vi "Timed Test.vi"() -> ()   [LabVIEW 2017]
uses:
  122af3c8-ed90-4da6-ba5e-d7198250e946.vi
  String Subset.vi
  Parsing/Parse Full Path or Item Name.vi
  Offset/Find Item Locations by Path.vi
  JSON text to Variant.vi
  JSONtext.lvlib
panel:
  out "time":dbl format="%#_3p"
  out "value":string
  out "Offsets":i32[](array[numeric])
  out "<JSON>":string[](array[string]) caption="<JSON>Items"
  out "Waveform Chart":dbl(graph)
  out "time/char":dbl format="%#_3p"
  out "Offset past Value":i32
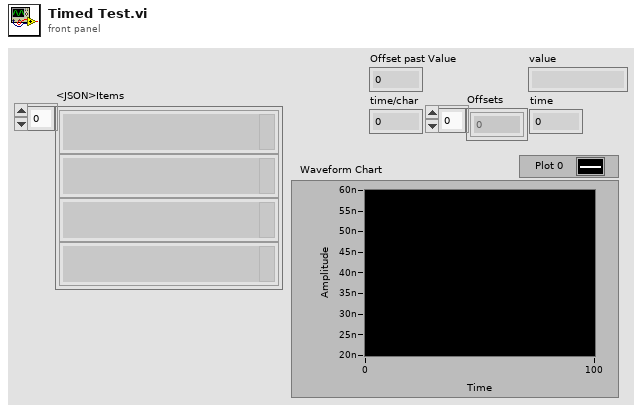
[diagram p1: front panel]
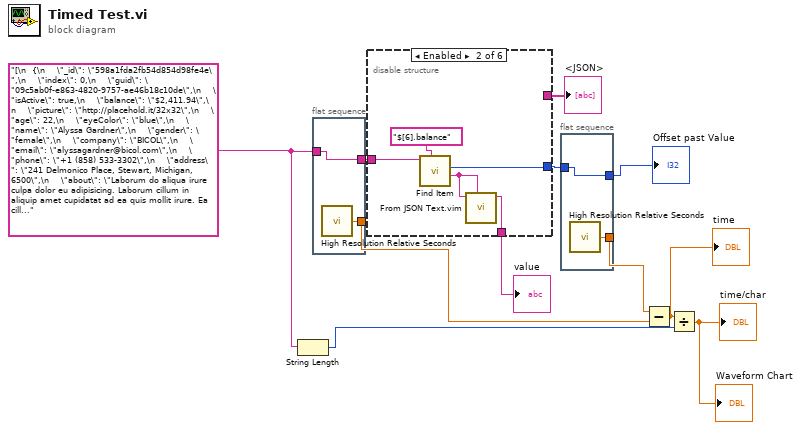
[diagram p0: block diagram]
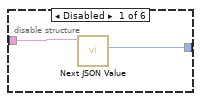
[diagram p2: hidden frame]
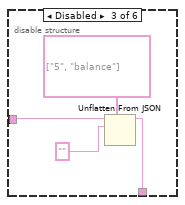
[diagram p3: hidden frame]
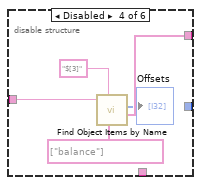
[diagram p4: hidden frame]
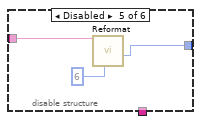
[diagram p5: hidden frame]
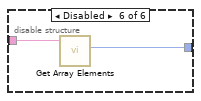
[diagram p6: hidden frame]
diagram:
  w6 = "[\n  {\n    \"_id\": \"598a1fda2fb54d854d98fe4e\",\n    \"index\": 0,\n    \"guid\": \"09c5ab0f-e863-4820-9757-ae46b18c10de\",\n    \"isActive\": true,\n    \"balance\": \"$2,411.94\",\n    \"picture\": \"http://placehold.it/32x32\",\n    \"age\": 22,\n    \"eyeColor\": \"blue\",\n    \"name\": \"Alyssa Gardner\",\n    \"gender\": \"female\",\n    \"company\": \"BICOL\",\n    \"email\": \"alyssagardner@bicol.com\",\n    \"phone\": \"+1 (858) 533-3302\",\n    \"address\": \"241 Delmonico Place, Stewart, Michigan, 6500\",\n    \"about\": \"Laborum do aliqua irure culpa dolor eu adipisicing. Laborum cillum in aliquip amet cupidatat ad ea quis mollit irure. Ea cillum exercitation nulla Lorem exercitation velit ad reprehenderit sint sint cupidatat elit reprehenderit. Incididunt aute tempor culpa ea sunt do sunt est deserunt deserunt eiusmod irure amet. Pariatur voluptate ea quis cupidatat non sit.\\r\\n\",\n    \"registered\": \"2016-12-13T10:56:52 -00:00\",\n    \"latitude\": -9.98155,\n    \"longitude\": -80.627111,\n    \"tags\": [\n      \"ad\",\n      \"cillum\",\n      \"est\",\n      \"et\",\n      \"deserunt\",\n      \"aliquip\",\n      \"cillum\"\n    ],\n    \"friends\": [\n      {\n        \"id\": 0,\n        \"name\": \"Karyn Weber\"\n      },\n      {\n        \"id\": 1,\n        \"name\": \"King Acevedo\"\n      },\n      {\n        \"id\": 2,\n        \"name\": \"Tanisha Rodgers\"\n      }\n    ],\n    \"greeting\": \"Hello, Alyssa Gardner! You have 6 unread messages.\",\n    \"favoriteFruit\": \"strawberry\"\n  },\n  {\n    \"_id\": \"598a1fda30b27ecb1964e718\",\n    \"index\": 1,\n    \"guid\": \"b7cddb7f-e542-4f41-b26c-7ddbecc986b3\",\n    \"isActive\": false,\n    \"balance\": \"$1,317.36\",\n    \"picture\": \"http://placehold.it/32x32\",\n    \"age\": 25,\n    \"eyeColor\": \"blue\",\n    \"name\": \"Skinner Andrews\",\n    \"gender\": \"male\",\n    \"company\": \"REMOLD\",\n    \"email\": \"skinnerandrews@remold.com\",\n    \"phone\": \"+1 (953) 523-2141\",\n    \"address\": \"515 Balfour Place, Gratton, Tennessee, 1793\",\n    \"about\": \"Nisi deserunt consectetur dolore reprehenderit ipsum dolore voluptate tempor nostrud est labore. Laborum ullamco do irure duis sunt sit quis consectetur dolore quis. Et veniam eu ad dolor. Anim incididunt tempor adipisicing elit veniam. Laboris esse amet pariatur pariatur aliqua ea dolore sunt dolor anim aliqua elit. Velit ipsum commodo deserunt esse aliquip sit.\\r\\n\",\n    \"registered\": \"2016-12-25T06:53:25 -00:00\",\n    \"latitude\": 72.774284,\n    \"longitude\": -22.688458,\n    \"tags\": [\n      \"dolore\",\n      \"nulla\",\n      \"deserunt\",\n      \"laboris\",\n      \"excepteur\",\n      \"eiusmod\",\n      \"ad\"\n    ],\n    \"friends\": [\n      {\n        \"id\": 0,\n        \"name\": \"Barron Rios\"\n      },\n      {\n        \"id\": 1,\n        \"name\": \"Roy Roy\"\n      },\n      {\n        \"id\": 2,\n        \"name\": \"Tonia Gates\"\n      }\n    ],\n    \"greeting\": \"Hello, Skinner Andrews! You have 5 unread messages.\",\n    \"favoriteFruit\": \"strawberry\"\n  },\n  {\n    \"_id\": \"598a1fdafd338fee73c75cc9\",\n    \"index\": 2,\n    \"guid\": \"e12f53e7-ffe2-40da-87a4-988a62c535d3\",\n    \"isActive\": true,\n    \"balance\": \"$3,792.67\",\n    \"picture\": \"http://placehold.it/32x32\",\n    \"age\": 21,\n    \"eyeColor\": \"green\",\n    \"name\": \"Lillie Spears\",\n    \"gender\": \"female\",\n    \"company\": \"KNEEDLES\",\n    \"email\": \"lilliespears@kneedles.com\",\n    \"phone\": \"+1 (946) 421-3701\",\n    \"address\": \"744 Dearborn Court, Brandywine, Massachusetts, 8302\",\n    \"about\": \"Dolor ad est cupidatat velit excepteur sunt. Id amet laborum nulla id magna deserunt nostrud et Lorem. Laboris amet tempor est cupidatat ullamco. Dolore Lorem aute duis quis sint in. Proident sunt laboris consectetur quis.\\r\\n\",\n    \"registered\": \"2016-01-29T12:32:53 -00:00\",\n    \"latitude\": -72.39395,\n    \"longitude\": -125.497614,\n    \"tags\": [\n      \"voluptate\",\n      \"sunt\",\n      \"et\",\n      \"amet\",\n      \"ea\",\n      \"anim\",\n      \"nisi\"\n    ],\n    \"friends\": [\n      {\n        \"id\": 0,\n        \"name\": \"Guzman Mcmahon\"\n      },\n      {\n        \"id\": 1,\n        \"name\": \"Craig Sampson\"\n      },\n      {\n        \"id\": 2,\n        \"name\": \"Gilliam Joseph\"\n      }\n    ],\n    \"greeting\": \"Hello, Lillie Spears! You have 5 unread messages.\",\n    \"favoriteFruit\": \"strawberry\"\n  },\n  {\n    \"_id\": \"598a1fdaae68ee444817bd5d\",\n    \"index\": 3,\n    \"guid\": \"896b1e41-bfd2-4e40-ac6f-ac9896540f87\",\n    \"isActive\": false,\n    \"balance\": \"$2,127.27\",\n    \"picture\": \"http://placehold.it/32x32\",\n    \"age\": 31,\n    \"eyeColor\": \"brown\",\n    \"name\": \"Massey Lopez\",\n    \"gender\": \"male\",\n    \"company\": \"BOLAX\",\n    \"email\": \"masseylopez@bolax.com\",\n    \"phone\": \"+1 (890) 530-3697\",\n    \"address\": \"130 National Drive, Eagleville, Oregon, 7451\",\n    \"about\": \"Excepteur elit consectetur Lorem occaecat culpa eu consequat reprehenderit dolore irure ullamco eiusmod mollit. Ut in aliquip dolor occaecat laborum officia veniam cillum. Consequat enim minim tempor culpa adipisicing et adipisicing aliqua esse minim fugiat. Magna in aute sint officia pariatur culpa. Labore exercitation quis laborum ipsum cillum incididunt dolor nostrud deserunt pariatur do sunt. Officia tempor consectetur sunt aliquip cillum nostrud do Lorem in. Sunt commodo minim officia nulla fugiat qui anim.\\r\\n\",\n    \"registered\": \"2016-06-20T11:25:17 -01:00\",\n    \"latitude\": -25.916761,\n    \"longitude\": -176.019318,\n    \"tags\": [\n      \"nisi\",\n      \"nisi\",\n      \"aliqua\",\n      \"nostrud\",\n      \"aliquip\",\n      \"mollit\",\n      \"cillum\"\n    ],\n    \"friends\": [\n      {\n        \"id\": 0,\n        \"name\": \"Florine Hubbard\"\n      },\n      {\n        \"id\": 1,\n        \"name\": \"Harper Peterson\"\n      },\n      {\n        \"id\": 2,\n        \"name\": \"Hayes Kaufman\"\n      }\n    ],\n    \"greeting\": \"Hello, Massey Lopez! You have 8 unread messages.\",\n    \"favoriteFruit\": \"banana\"\n  },\n  {\n    \"_id\": \"598a1fda5ee0d6fed3630e62\",\n    \"index\": 4,\n    \"guid\": \"8e1a25a0-83eb-45b2-9e18-c4b03a903295\",\n    \"isActive\": true,\n    \"balance\": \"$1,882.49\",\n    \"picture\": \"http://placehold.it/32x32\",\n    \"age\": 26,\n    \"eyeColor\": \"brown\",\n    \"name\": \"Ginger Black\",\n    \"gender\": \"female\",\n    \"company\": \"KROG\",\n    \"email\": \"gingerblack@krog.com\",\n    \"phone\": \"+1 (924) 450-3688\",\n    \"address\": \"843 Jackson Place, Greenwich, Puerto Rico, 8966\",\n    \"about\": \"Nostrud tempor quis elit nulla consectetur. Reprehenderit voluptate enim ea aliquip minim commodo proident ipsum commodo ex. Commodo nisi nulla magna amet. Officia minim cillum minim nostrud eiusmod tempor ut cillum cillum culpa. Non do reprehenderit esse consectetur aliquip. Ipsum excepteur esse veniam id nulla sunt enim nulla reprehenderit elit non reprehenderit fugiat dolore.\\r\\n\",\n    \"registered\": \"2016-03-21T08:14:28 -00:00\",\n    \"latitude\": 16.438889,\n    \"longitude\": -11.148876,\n    \"tags\": [\n      \"commodo\",\n      \"ipsum\",\n      \"exercitation\",\n      \"est\",\n      \"culpa\",\n      \"do\",\n      \"anim\"\n    ],\n    \"friends\": [\n      {\n        \"id\": 0,\n        \"name\": \"Taylor Ball\"\n      },\n      {\n        \"id\": 1,\n        \"name\": \"Irma Guerrero\"\n      },\n      {\n        \"id\": 2,\n        \"name\": \"Allison Fitzpatrick\"\n      }\n    ],\n    \"greeting\": \"Hello, Ginger Black! You have 6 unread messages.\",\n    \"favoriteFruit\": \"strawberry\"\n  },\n  {\n    \"_id\": \"598a1fdab7c3311e6bd5eb22\",\n    \"index\": 5,\n    \"guid\": \"81b72db8-8d6a-4430-a934-c8454fbade9b\",\n    \"isActive\": true,\n    \"balance\": \"$2,347.48\",\n    \"picture\": \"http://placehold.it/32x32\",\n    \"age\": 23,\n    \"eyeColor\": \"blue\",\n    \"name\": \"Hobbs Rocha\",\n    \"gender\": \"male\",\n    \"company\": \"FARMEX\",\n    \"email\": \"hobbsrocha@farmex.com\",\n    \"phone\": \"+1 (904) 467-2057\",\n    \"address\": \"982 Forrest Street, Moquino, Utah, 6900\",\n    \"about\": \"Nulla et proident ullamco cupidatat quis nisi officia. Duis nulla proident ullamco consectetur ut dolore sint tempor ex. Ut consequat consequat sint ipsum est esse aliquip ullamco cupidatat ea.\\r\\n\",\n    \"registered\": \"2016-10-22T12:39:06 -01:00\",\n    \"latitude\": 40.819623,\n    \"longitude\": -115.648188,\n    \"tags\": [\n      \"duis\",\n      \"sunt\",\n      \"cillum\",\n      \"ex\",\n      \"qui\",\n      \"Lorem\",\n      \"esse\"\n    ],\n    \"friends\": [\n      {\n        \"id\": 0,\n        \"name\": \"Louella Cantrell\"\n      },\n      {\n        \"id\": 1,\n        \"name\": \"Franklin Hunt\"\n      },\n      {\n        \"id\": 2,\n        \"name\": \"Randolph Bruce\"\n      }\n    ],\n    \"greeting\": \"Hello, Hobbs Rocha! You have 5 unread messages.\",\n    \"favoriteFruit\": \"strawberry\"\n  },\n  {\n    \"_id\": \"598a1fda52128973d4b98281\",\n    \"index\": 6,\n    \"guid\": \"0ef2d183-da74-43c8-82bf-f8f5655bcaf2\",\n    \"isActive\": false,\n    \"balance\": \"$1,064.96\",\n    \"picture\": \"http://placehold.it/32x32\",\n    \"age\": 23,\n    \"eyeColor\": \"brown\",\n    \"name\": \"Meghan Barlow\",\n    \"gender\": \"female\",\n    \"company\": \"IMMUNICS\",\n    \"email\": \"meghanbarlow@immunics.com\",\n    \"phone\": \"+1 (947) 482-3495\",\n    \"address\": \"356 Mill Road, Keyport, Alabama, 8120\",\n    \"about\": \"Lorem pariatur Lorem sint mollit Lorem et deserunt consectetur pariatur laborum voluptate occaecat laboris nulla. Aliqua duis esse cupidatat cupidatat pariatur excepteur do duis duis do qui. Fugiat mollit exercitation consectetur et tempor labore tempor. Aute magna commodo ut culpa deserunt laboris duis cillum minim.\\r\\n\",\n    \"registered\": \"2015-02-01T10:42:34 -00:00\",\n    \"latitude\": -36.45445,\n    \"longitude\": -148.168895,\n    \"tags\": [\n      \"in\",\n      \"id\",\n      \"irure\",\n      \"proident\",\n      \"aliquip\",\n      \"cupidatat\",\n      \"magna\"\n    ],\n    \"friends\": [\n      {\n        \"id\": 0,\n        \"name\": \"Sellers Garcia\"\n      },\n      {\n        \"id\": 1,\n        \"name\": \"Maureen Leonard\"\n      },\n      {\n        \"id\": 2,\n        \"name\": \"Sparks Page\"\n      }\n    ],\n    \"greeting\": \"Hello, Meghan Barlow! You have 2 unread messages.\",\n    \"favoriteFruit\": \"banana\"\n  }\n]" ("JSON")
  n1 = String Length(string=w6) -> (length=w5:i32)
  n2 = flat-sequence {
    tunnel: [w13] -> w11
    tunnel: w6 -> [w13]
    tunnel: [w12] -> w7
    frame #0 {
      n3 = call <vilib>:"High Resolution Relative Seconds.vi"() -> ("relative seconds"=w12:dbl)
    }
  }
  n4 = disable-structure shown="Enabled" {
    disable-tunnel: w11 -> [w15 w20 w24 w29 w32 w34]
    disable-tunnel: [w14 w19 _ _ w31 w33] -> w10
    disable-tunnel: [_ _ _ w26 _ _] -> w3
    disable-tunnel: [_ w16 w21 _ _ _] -> w2
    frame Disabled {
      n5 = call "Next JSON Value.vi"("JSON"=w15) -> ("Offset past"=w14:i32)  [unwired: 7 in, 3 out]
    }
    frame Enabled {
      n6 = call "Find Item.vi"("$Path or Item Name"="$[6].balance", "JSON"=w20) -> ("<JSON>"=w17:string, "Item offset"=w19:i32)  [unwired: 6 in, 2 out]
      n7 = call "From JSON Text.vim"("Data Type and Default Value"=w17, "JSON"=w17) -> ("Data out"=w16:string)  [unwired: 8 in, 1 out]
    }
    frame Disabled {
      n8 = Unflatten From JSON(path=string[] ["5", "balance"], JSON string=w24, type and defaults="") -> (value=w21:string)  [unwired: 4 in, 1 out]
    }
    frame Disabled {
      n9 = call "Find Object Items by Name.vi"("Item Names"=string[] ["balance"], "$Path or Item Name"="$[3]" ("Object Path"), "JSON"=w29) -> ("<JSON>"=w26:string[], "Offsets"=→"Offsets":i32[])  [unwired: 6 in, 1 out]
    }
    frame Disabled {
      n10 = call "Reformat.vi"("Pretty Print Levels"=6, "JSON"=w32) -> ("Offset past"=w31:i32)  [unwired: 6 in, 3 out]
    }
    frame Disabled {
      n11 = call "Get Array Elements.vi"("JSON"=w34) -> ("Offset past"=w33:i32)  [unwired: 8 in, 2 out]
    }
  }
  "<JSON>" <- w3
  "value" <- w2
  n12 = flat-sequence {
    tunnel: [w36] -> w9
    tunnel: w10 -> [w36]
    tunnel: [w35] -> w8
    frame #0 {
      n13 = call <vilib>:"High Resolution Relative Seconds.vi"() -> ("relative seconds"=w35:dbl)
    }
  }
  n14 = Subtract(x=w8, y=w7) -> (x-y=w1:dbl)
  "time" <- w1
  n15 = Divide(x=w1, y=w5) -> (x/y=→"time/char" →"Waveform Chart":dbl)
  "Offset past Value" <- w9
